vi "Set Static (Global).vi"(8 "error in (no error)":errorcluster, 10 "Int":i32, 11 "Numeric in":refnum<class "Numeric Test Object.lvclass">) -> (0 "error out":errorcluster, 3 "Numeric out":refnum<class "Numeric Test Object.lvclass">)   [LabVIEW 2009, in "Numeric Test Object.lvclass"]
doc: "Sets the data held by the global variable."
uses:
  Numeric Test Object.lvclass
  _Static Data (Global).vi
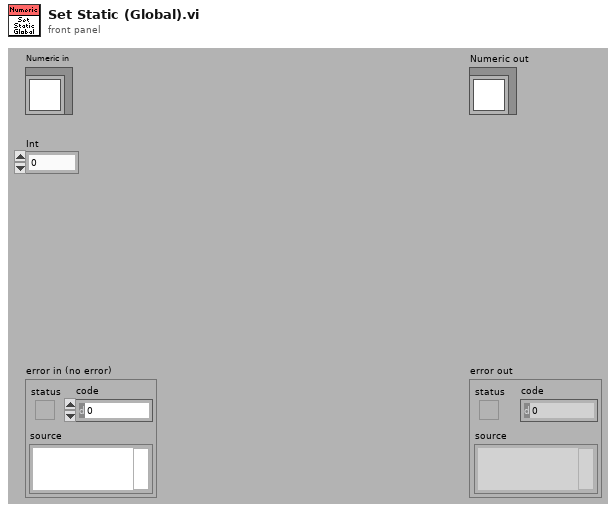
[diagram p1: front panel]
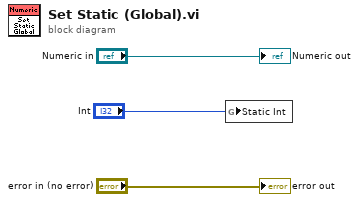
[diagram p0: block diagram]
diagram:
  n1 = global write "_Static Data (Global).vi" "Static Int"("Int") -> ()
  "error out" <- "error in (no error)"
  "Numeric out" <- "Numeric in"
